vi "Handle M12.vi"(0 "reference in":refnum<class "PM_Group.lvclass">, 11 "error in (no error)":errorcluster) -> (4 "reference out":refnum<class "PM_Group.lvclass">, 15 "error out":errorcluster)   [LabVIEW 2019, in "PM_Group.lvclass"]
uses:
  PM_Group.lvclass
  FPGA/TypeDef/AI index.ctl
  PM_Group.lvclass/PM_Group.ctl
  AI_class/AI.lvclass/AI.ctl
  AnalogComparator_class/AnalogComparator.lvclass/AnalogComparator.ctl
  TypeDef/State Engine.ctl
  Device_class/Device.lvclass/Device.ctl
  Engine_1DO_2DI_class/Engine_1DO_2DI.lvclass/Engine_1DO_2DI.ctl
  AnalogComparator_class/GetStatus.vi
  Device_class/GetFPGA.vi
  Engine_1DO_2DI_class/Engine_1DO_2DI.lvclass
  C:/Users/ANENKOV_V1/Desktop/src/Device_class/Device.lvclass
  FPGA_API_class/FPGA API.lvclass
  AI_class/AI.lvclass
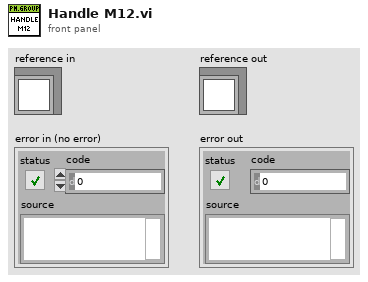
[diagram p1: front panel]
types:
  T1 = typedef "AI index.ctl" = u8
  T2 = typedef "AI_Data.ctl" = cluster{"Stat Data":T3, "OutOfRangeMax":bool, "OutOfRangeMin":bool, "HIHI":bool, "HI":bool, "LO":bool, "LOLO":bool}
  T3 = typedef "AI Statistics Data.ctl" = cluster{"raw mean":dbl, "scl mean":dbl, "raw mean 1Hz":dbl, "scl mean 1Hz":dbl}
  T4 = typedef "State Engine.ctl" = enum16{"Unknown", "Off", "TupningOn", "On", "TurningOff"}
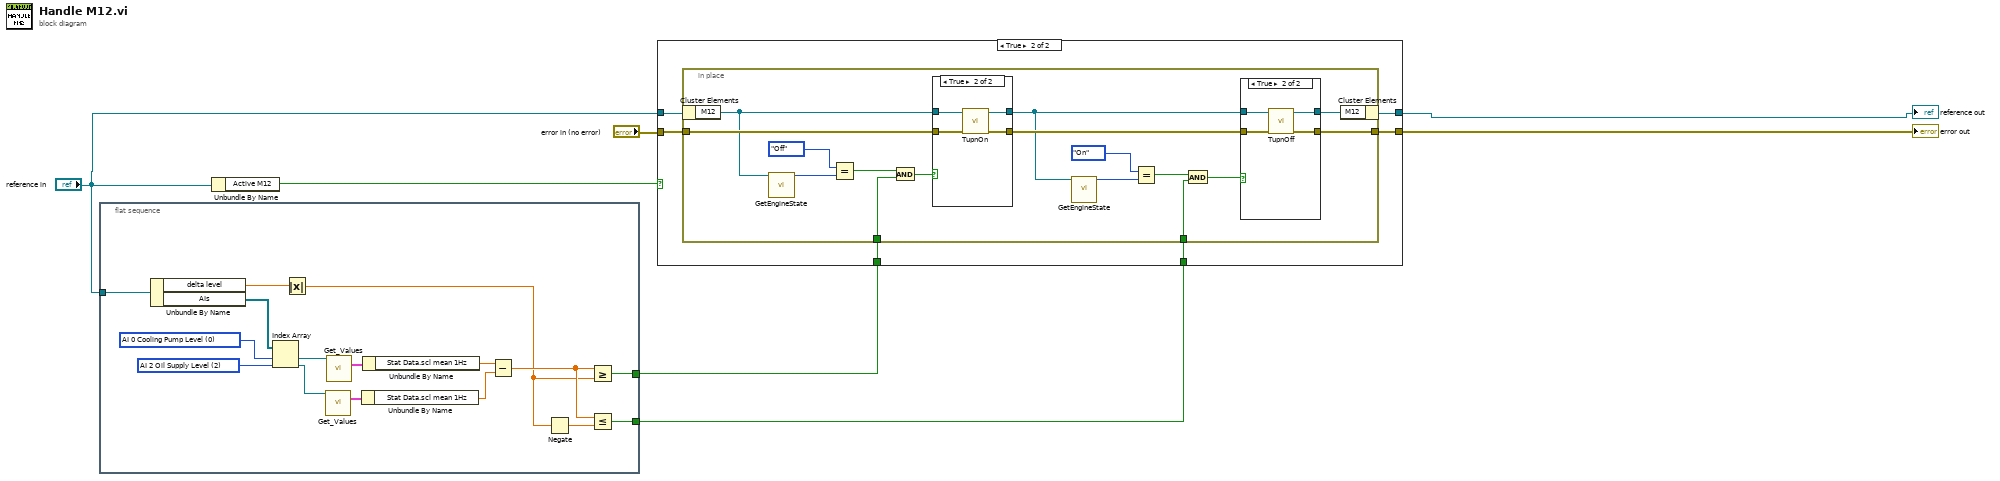
[diagram p0: block diagram]
diagram:
  n1 = flat-sequence {
    tunnel: "reference in" -> [w18]
    tunnel: [w12] -> w2
    tunnel: [w8] -> w1
    frame #0 {
      w21 = T1 2 items=["AI 0 Cooling Pump Level", "AI 1 Cooling Pump Temp", "AI 2 Oil Supply Level", "AI 3 Oil Supply Temp", "AI 4 ", "AI 5 Pressure Haskel", "AI 6 Pressure DUT", "AI 7 Pressure Chamber", "AI 8 Pressure Air inlet", "AI 9 Pressure Air outlet", "AI 10 Pressure Messure Line"] ("AI index")
      w19 = T1 0 items=["AI 0 Cooling Pump Level", "AI 1 Cooling Pump Temp", "AI 2 Oil Supply Level", "AI 3 Oil Supply Temp", "AI 4 ", "AI 5 Pressure Haskel", "AI 6 Pressure DUT", "AI 7 Pressure Chamber", "AI 8 Pressure Air inlet", "AI 9 Pressure Air outlet", "AI 10 Pressure Messure Line"] ("AI index")
      n2 = Unbundle By Name(w18) -> ("delta level"=w13:dbl, "AIs"=w20:refnum<class "AI.lvclass">[])
      n3 = Index Array(array=w20, index #1=w19, index #2=w21) -> (element #1=w17:refnum<class "AI.lvclass">, element #2=w16:refnum<class "AI.lvclass">)
      n4 = Absolute Value(x=w13) -> (abs(x)=w9:dbl)
      n5 = call "Get_Values.vi"("reference in"=w16) -> ("Data"=w23:T2)  [unwired: 14 in]
      n6 = call "Get_Values.vi"("reference in"=w17) -> ("Data"=w22:T2)  [unwired: 14 in]
      n7 = Unbundle By Name(w23) -> ("Stat Data.scl mean 1Hz"=w15:dbl)
      n8 = Unbundle By Name(w22) -> ("Stat Data.scl mean 1Hz"=w14:dbl)
      n9 = Subtract(x=w14, y=w15) -> (x-y=w11:dbl)
      n10 = Negate(x=w9) -> (-x=w10:dbl)
      n11 = Greater Or Equal?(x=w11, y=w9) -> (x >= y?=w12:bool)
      n12 = Less Or Equal?(x=w11, y=w10) -> (x <= y?=w8:bool)
    }
  }
  n13 = Unbundle By Name("reference in") -> ("Active M12"=w7:bool)
  n14 = case shown="True" w7 {
    tunnel: [w25 w31] -> w4
    tunnel: [w24 w30] -> w3
    tunnel: "reference in" -> [w25 w29]
    tunnel: "error in (no error)" -> [w24 w28]
    tunnel: w2 -> [_ w27]
    tunnel: w1 -> [_ w26]
    frame False {
    }
    frame True {
      n15 = in-place {
        in-place-border: w28 -> [w44]
        in-place-border: [w41] -> w30
        in-place-border: w27 -> [w33]
        in-place-border: w26 -> [w32]
        n16 = in-place-cluster #1(w29) -> ("M12"=w43:refnum<class "Engine_1DO_2DI.lvclass">)
        n17 = call "GetEngineState.vi"("Engine"=w43) -> ("EngineState"=w46:T4)  [unwired: 10 in, 4 out]
        n18 = Equal?(x=State_Engine."Off" ("y"), y=w46) -> (x = y?=w40:bool)
        n19 = Compound Arithmetic op=AND(w40, w33) -> (w39:bool)
        n20 = case shown="True" w39 {
          tunnel: w44 -> [w48 w53]
          tunnel: w43 -> [w49 w52]
          tunnel: [w49 w51] -> w36
          tunnel: [w48 w50] -> w42
          frame False {
          }
          frame True {
            n21 = call "TupnOn.vi"("error in (no error)"=w53, "Pump_1AI_1DO_2DI in"=w52) -> ("error out"=w50:errorcluster, "Pump_1AI_1DO_2DI out"=w51:refnum<class "Engine_1DO_2DI.lvclass">)  [unwired: 8 in]
          }
        }
        n22 = call "GetEngineState.vi"("Engine"=w36) -> ("EngineState"=w38:T4)  [unwired: 10 in, 4 out]
        n23 = Equal?(x=State_Engine."On" ("y"), y=w38) -> (x = y?=w35:bool)
        n24 = And(x=w35, y=w32) -> (x .and. y?=w34:bool)
        n25 = case shown="True" w34 {
          tunnel: w36 -> [w54 w59]
          tunnel: [w54 w58] -> w45
          tunnel: w42 -> [w55 w57]
          tunnel: [w55 w56] -> w41
          frame False {
          }
          frame True {
            n26 = call "TupnOff.vi"("error in (no error)"=w57, "Pump_1AI_1DO_2DI in"=w59) -> ("error out"=w56:errorcluster, "Pump_1AI_1DO_2DI out"=w58:refnum<class "Engine_1DO_2DI.lvclass">)  [unwired: 8 in]
          }
        }
        n27 = in-place-cluster #1("M12"=w45) -> (w31:refnum<class "PM_Group.lvclass">)
      }
    }
  }
  "error out" <- w3
  "reference out" <- w4
